vi "3.0-The Timing Badass.vi"(1 "Start":u32, 2 "End":u32) -> (0 "Super Heart Beat":T1)   [LabVIEW 2010]
uses:
  4-High Neurons/4.0-Timing Badass.ctl
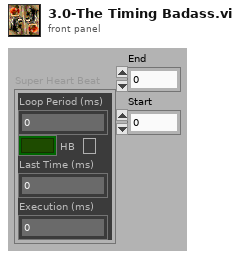
[diagram p1: front panel]
types:
  T1 = typedef "4.0-Timing Badass.ctl" = cluster{"Loop Period (ms)":u32, "HB":bool, "Last Time (ms)":u32, "Execution (ms)":u32}
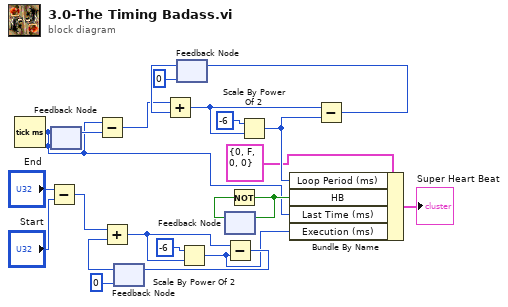
[diagram p0: block diagram]
diagram:
  n1 = Tick Count (ms)() -> (millisecond timer value=w13:u32)
  n2 = Subtract(x="End", y="Start") -> (x-y=w4:u32)
  n3 = feedback #1(w13) -> (w22:u32)
  n4 = feedback-in #1(w13) -> ()
  n5 = Subtract(x=w13, y=w22) -> (x-y=w15:u32)
  n6 = feedback #2(u32 0) -> (w6:u32)
  n7 = Add(x=w4, y=w6) -> (x+y=w7:u32)
  n8 = feedback #3(u32 0) -> (w21:u32)
  n9 = Add(x=w15, y=w21) -> (x+y=w20:u32)
  n10 = Scale By Power Of 2(n=-6, x=w7) -> (x*2^n=w1:u32)
  n11 = feedback #4() -> (w17:bool)  [unwired: 1 in]
  n12 = Subtract(x=w7, y=w1) -> (x-y=w5:u32)
  n13 = feedback-in #2(w5) -> ()
  n14 = Not(x=w17) -> (.not. x?=w16:bool)
  n15 = feedback-in #4(w16) -> ()
  n16 = Scale By Power Of 2(n=-6, x=w20) -> (x*2^n=w12:u32)
  n17 = Bundle By Name(cluster=T1 {"Loop Period (ms)"=0, "HB"=FALSE, "Last Time (ms)"=0, "Execution (ms)"=0} ("Loop Update Cluster"), "Loop Period (ms)"=w12, "HB"=w16, "Last Time (ms)"=w13, "Execution (ms)"=w1) -> (→"Super Heart Beat":T1)
  n18 = Subtract(x=w20, y=w12) -> (x-y=w19:u32)
  n19 = feedback-in #3(w19) -> ()
